vi "SHSW Specific Heat Correlation of Saline Water (J to Kg to K).vi"(1 "Salinity":dbl, 2 "Sailne Water Temprature":dbl[unit]) -> (0 "SHSW":dbl[unit])   [LabVIEW 2018]
panel:
  out "Temprature Of Saline Water\nKelvin Degree":dbl[unit](slide) scale=273.0..373.0
  out "Tk":dbl[unit]
  out "Saline Water Temprature":dbl[unit](slide) scale=0.0..100.0
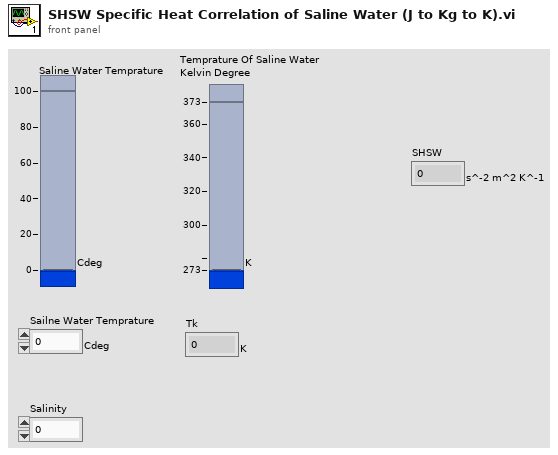
[diagram p1: front panel]
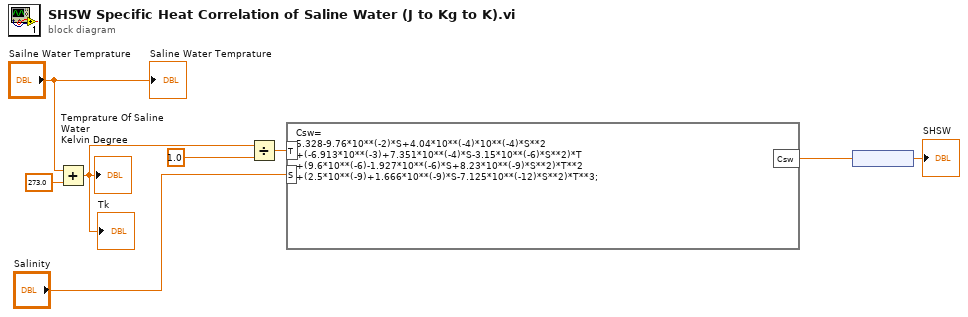
[diagram p0: block diagram]
diagram:
  n1 = Add(x="Sailne Water Temprature", y=dbl[unit] 273.0) -> (x+y=w2:dbl[unit])
  "Tk" <- w2
  "Temprature Of Saline Water\nKelvin Degree" <- w2
  n2 = Divide(x=w2, y=dbl[unit] 1.0) -> (x/y=w8:dbl)
  n3 = formula code="Csw=\n5.328-9.76*10**(-2)*S+4.04*10**(-4)*10**(-4)*S**2\n+(-6.913*10**(-3)+7.351*10**(-4)*S-3.15*10**(-6)*S**2)*T\n+(9.6*10**(-6)-1.927*10**(-6)*S+8.23*10**(-9)*S**2)*T**2\n+(2.5*10**(-9)+1.666*10**(-9)*S-7.125*10**(-12)*S**2)*T**3;"("T"=w8, "S"="Salinity") -> ("Csw"=w6:dbl)
  n4 = node(w6) -> (→"SHSW":dbl[unit])
  "Saline Water Temprature" <- "Sailne Water Temprature"
